vi "IndoorData_GetInstance.vi"(0 "reference in":refnum<class "IndoorData.lvclass"> caption="This control should only be used when\na sub class is inheriting this class", 5 "error in (no error)":errorcluster) -> (12 "ObjectQueueName":string caption="This queue name could be used to destroy\nthe named queue that is used to hold the\nreference in the clean up.", 14 "reference out":refnum<class "IndoorData.lvclass"> caption="This indicator should only be used when\na sub class is inheriting this class", 15 "NewObjectCreated":bool, 16 "DVRRefOut":refnum<data-value>, 19 "error out":errorcluster)   [LabVIEW 2014, in "IndoorData.lvclass"]
uses:
  IndoorData.lvclass
  ObjectAttributes.ctl
  DebugData.ctl
  ActualValues.ctl
  BufferedReadings.ctl
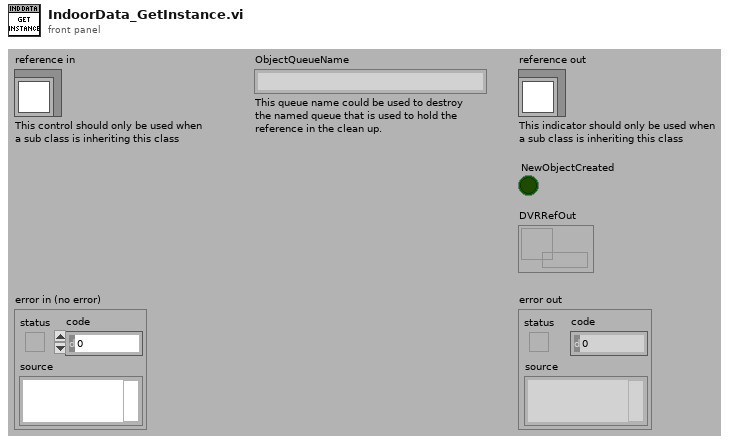
[diagram p1: front panel]
types:
  T1 = enum16{"Create or look up existing", "Look up existing"}
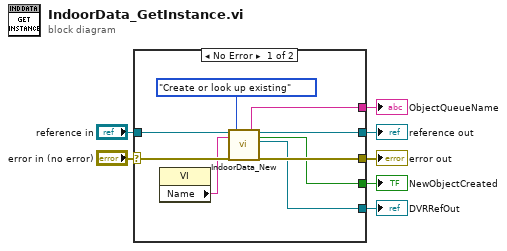
[diagram p0: block diagram]
diagram:
  n1 = case shown="No Error" "error in (no error)" {
    selector: "error in (no error)" -> [w15 w18]
    tunnel: [w16 w17] -> w7
    tunnel: [w14 w18] -> w5
    tunnel: "reference in" -> [w12 w17]
    tunnel: [w11 _] -> w3
    tunnel: [w10 _] -> w2
    tunnel: [w8 _] -> w1
    frame No Error {
      n2 = property class="VI"() -> ("Name"=w13:string)  [unwired: 2 in, 2 out]
      n3 = call "IndoorData_New.vi"("reference in"=w12, "Object name"=w13, "error in (no error)"=w15, "CreateMethod(Create or look up existing)"=T1."Create or look up existing") -> ("ObjectQueueName"=w8:string, "reference out"=w16:refnum<class "IndoorData.lvclass">, "NewObjectCreated"=w11:bool, "DVRRefOut"=w10:refnum<data-value>, "error out"=w14:errorcluster)  [unwired: 11 in]
    }
    frame Error {
    }
  }
  "reference out" <- w7
  "error out" <- w5
  "NewObjectCreated" <- w3
  "DVRRefOut" <- w2
  "ObjectQueueName" <- w1
